vi "Pre-Build VI - Run Unit Tests.vi"(8 "error in (no error)":errorcluster) -> (0 "error out":errorcluster, 1 "VIs without test coverage":string[](array[string]), 2 "error type":enum16{"fatal", "non-fatal", "warning"}(ring))   [LabVIEW 2009]
uses:
  <userlib>/_OpenG.lib/array/array.llb/Filter 1D Array (String)__ogtk.vi
panel:
  in  "type specifier VI Refnum (for type only)":refnum<vi>
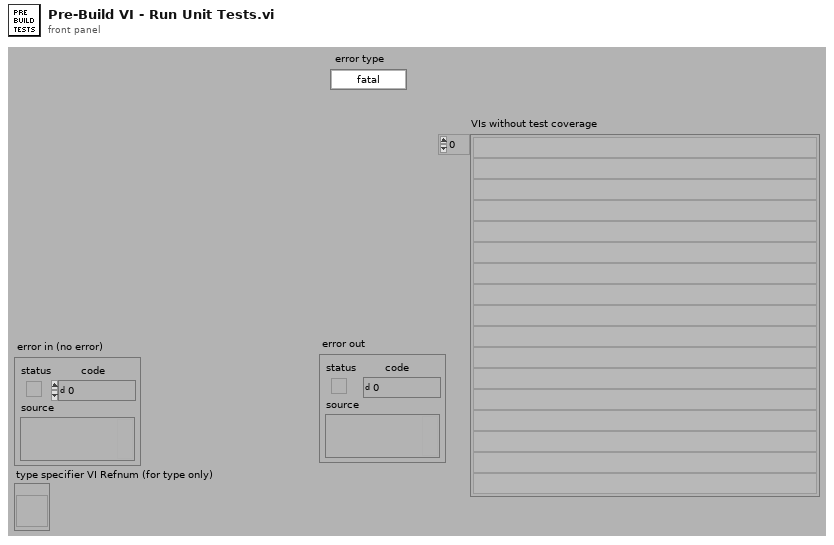
[diagram p1: front panel]
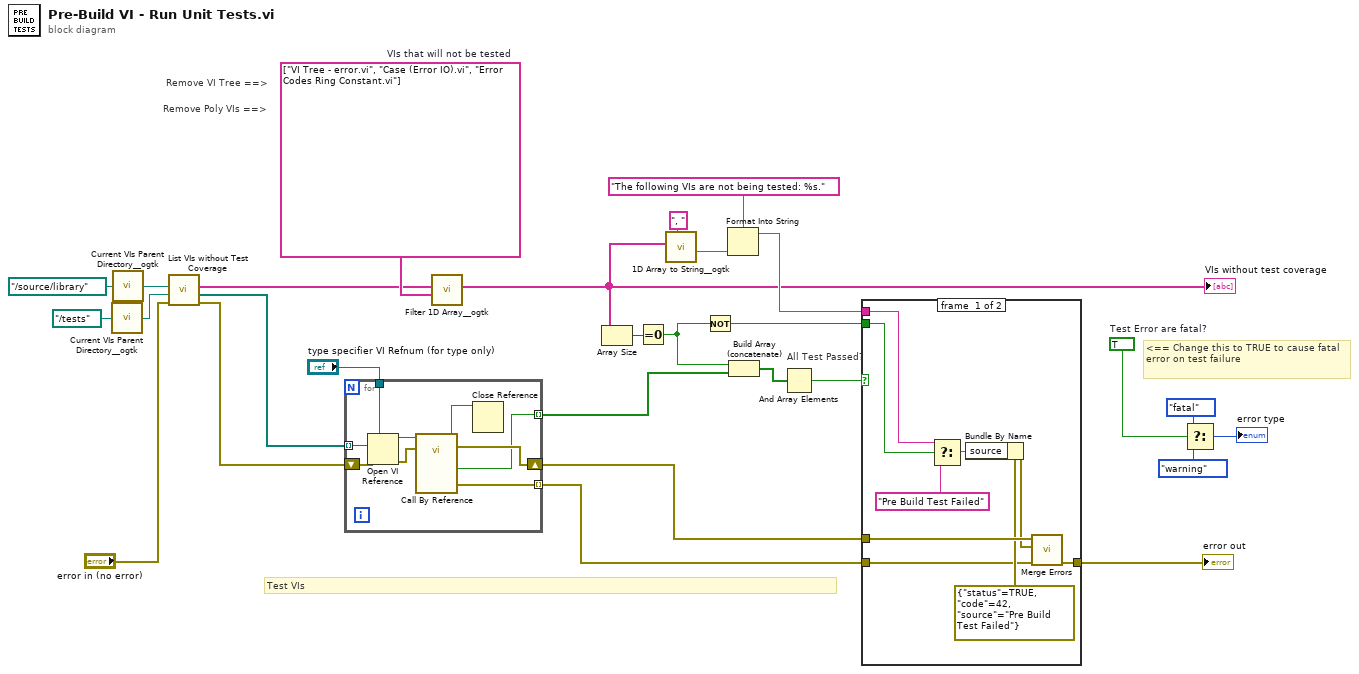
[diagram p0: block diagram]
diagram:
  w15 = TRUE  # Test Error are fatal?
  w26 = string[] ["VI Tree - error.vi", "Case (Error IO).vi", "Error Codes Ring Constant.vi"]  # VIs that will not be tested
  # "<== Change this to TRUE to cause fatal error on test failure"
  # "Remove Poly VIs ==>"
  # "Remove VI Tree ==>"
  # "All Test Passed?"
  # "Test VIs"
  n1 = call <userlib>:"Current VIs Parent Directory__ogtk.vi"("Relative path (.)"=path "../tests") -> ("Parent Directory (+ Relative)"=w10:path)  [unwired: 4 in]
  n2 = call <userlib>:"Current VIs Parent Directory__ogtk.vi"("Relative path (.)"=path "../source/library") -> ("Parent Directory (+ Relative)"=w19:path)  [unwired: 4 in]
  n3 = call "List VIs without Test Coverage.vi"("error in (no error)"="error in (no error)", "Tests Root"=w10, "Source Root"=w19) -> ("error out"=w6:errorcluster, "Test VIs"=w9:path[], "VIs without test coverage"=w25:string[])  [unwired: 6 in]
  n4 = for {
    tunnel: w9 -> [w37] mode=indexing
    tunnel: "type specifier VI Refnum (for type only)" -> [w36]
    shift-right: [w33] -> w7
    shift-left: w6 -> [w32]
    tunnel: [w31] -> w5 mode=indexing
    tunnel: [w29] -> w4 mode=indexing
    n5 = Open VI Reference(type specifier VI Refnum (for type only)=w36, vi path=w37, error in (no error)=w32) -> (vi reference=w35:refnum<vi>, error out=w34:errorcluster)  [unwired: 3 in]
    n6 = call-by-ref "?"(reference=w35, error in=w34) -> (reference out=w30:refnum<vi>, error out=w33:errorcluster, 0:"error out"=w29:errorcluster, "pass"=w31:bool)  [unwired: 10 in]
    n7 = Close Reference(reference=w30) -> ()  [unwired: 1 in, 1 out]
  }
  n8 = call-poly <userlib>:"Filter 1D Array__ogtk.vi"("items to filter"=w26, "array"=w25) -> ("filtered array"=w3:string[])  [unwired: 4 in, 1 out]
  "VIs without test coverage" <- w3
  n9 = Array Size(array=w3) -> (size(s)=w2:i32)
  n10 = Equal To 0?(x=w2) -> (x = 0?=w1:bool)
  n11 = call <userlib>:"1D Array to String__ogtk.vi"("delimiter (Tab)"=", ", "Array of Strings"=w3) -> ("delimited string"=w23:string)  [unwired: 9 in]
  n12 = Not(x=w1) -> (.not. x?=w20:bool)
  n13 = Format Into String(format string="The following VIs are not being tested: %s.", w23) -> (resulting string=w21:string)  [unwired: 2 in, 1 out]
  n14 = Build Array (concatenate)(w1, w5) -> (w28:bool[])
  n15 = And Array Elements(Boolean array=w28) -> (logical AND=w27:bool)
  n16 = case shown="False" w27 {
    tunnel: w7 -> [w46 w47]
    tunnel: [w45 w47] -> w17
    tunnel: w20 -> [w44 _]
    tunnel: w21 -> [w43 _]
    tunnel: w4 -> [w38 _]
    frame #0 {
      n17 = Select(t=w43, s=w44, f="Pre Build Test Failed" ("source")) -> (s? t:f=w41:string)
      n18 = Bundle By Name(cluster=errorcluster {"status"=TRUE, "code"=42, "source"="Pre Build Test Failed"} ("error out"), "source"=w41) -> (w40:errorcluster)
      n19 = call <vilib>:"Merge Errors.vi"("error array in"=w38, "error in 2 (no error)"=w40, "error in 1 (no error)"=w46) -> ("error out"=w45:errorcluster)  [unwired: 4 in]
    }
    frame #1 {
    }
  }
  "error out" <- w17
  n20 = Select(t=enum16{"fatal", "non-fatal", "warning"}."fatal" ("error type"), s=w15, f=enum16{"fatal", "non-fatal", "warning"}."warning" ("error type")) -> (s? t:f=→"error type":enum16{"fatal", "non-fatal", "warning"})
